vi "Configure Input Signal.vi"(6 "Input Notch Filter (0: None)":u16(ring) items=["None", "Line Notch", "2x Line Notch", "Both Notch Filters"], 7 "Input Shield Grounding (0: Float)":u16(ring) items=["Float", "Ground"], 8 "error in (no error)":errorcluster, 9 "Input Coupling (0: AC)":u16(ring) items=["AC", "DC"], 10 "Input Connection (0: Single-Ended Voltage)":u16(ring) items=["Single-Ended Voltage", "Differential Voltage", "1 MOhm Current Gain", "100 MOhm Current Gain"], 11 "VISA resource name":refnum<visa-resource-name>) -> (0 "error out":errorcluster, 3 "VISA resource name out":refnum<visa-resource-name>)   [LabVIEW 2016, in "Stanford Research 830.lvlib"]
doc: "Configures the required input signal parameters."
uses:
  Stanford Research 830.lvlib
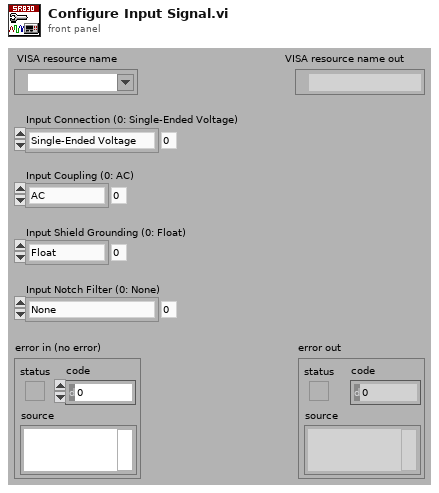
[diagram p1: front panel]
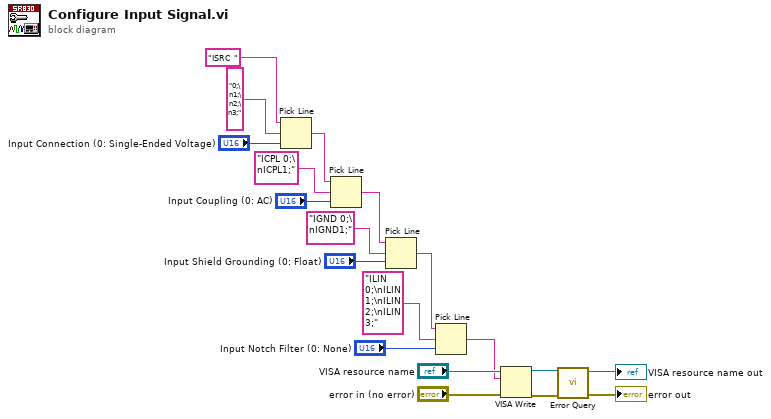
[diagram p0: block diagram]
diagram:
  n1 = Pick Line(string ("")="ISRC ", multi-line string="0;\n1;\n2;\n3;", line index="Input Connection (0: Single-Ended Voltage)") -> (output string=w13:string)
  n2 = Pick Line(string ("")=w13, multi-line string="ICPL 0;\nICPL1;", line index="Input Coupling (0: AC)") -> (output string=w10:string)
  n3 = Pick Line(string ("")=w10, multi-line string="IGND 0;\nIGND1;", line index="Input Shield Grounding (0: Float)") -> (output string=w8:string)
  n4 = Pick Line(string ("")=w8, multi-line string="ILIN 0;\nILIN 1;\nILIN 2;\nILIN 3;", line index="Input Notch Filter (0: None)") -> (output string=w5:string)
  n5 = VISA Write(VISA resource name="VISA resource name", write buffer=w5, error in (no error)="error in (no error)") -> (VISA resource name out=w4:refnum<visa-resource-name>, error out=w1:errorcluster)  [unwired: 1 out]
  n6 = call "Error Query.vi"("error in (no error)"=w1, "VISA resource name"=w4) -> ("error out"=→"error out":errorcluster, "VISA resource name out"=→"VISA resource name out":refnum<visa-resource-name>)  [unwired: 7 in, 1 out]
